vi "mean bulid.vi"(6 "reset data":bool, 8 "mean factor":dbl=-40.0 format="%#_13g", 9 "channel":dbl, 10 "new data":T2, 11 "memory data":T1(array[cluster])) -> (0 "amp cal":cluster{"freqency":dbl[], "Array":dbl[]}, 1 "phase cal":cluster{"freqency":dbl[], "Array":dbl[]}, 3 "memory data":T1(array[cluster]))   [LabVIEW 2021]
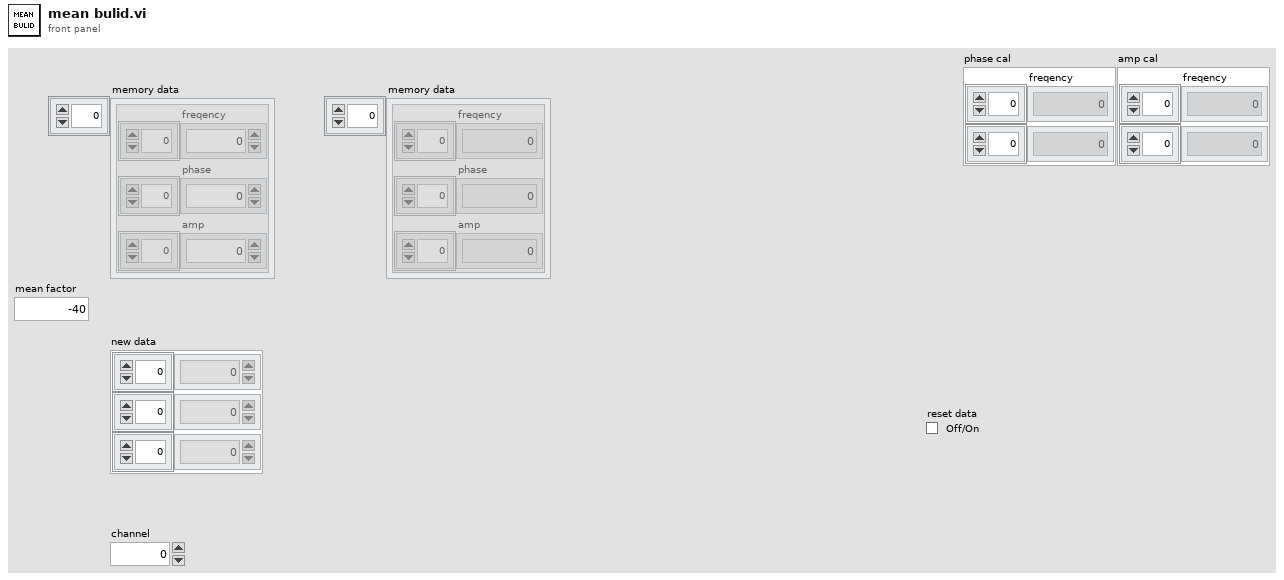
[diagram p1: front panel]
types:
  T1 = cluster{"freqency":dbl[], "phase":dbl[], "amp":dbl[]}[]
  T2 = cluster{"Array":dbl[], "Array":dbl[], "Array":dbl[]}
  T3 = cluster{"freqency":dbl[], "phase":dbl[], "amp":dbl[]}
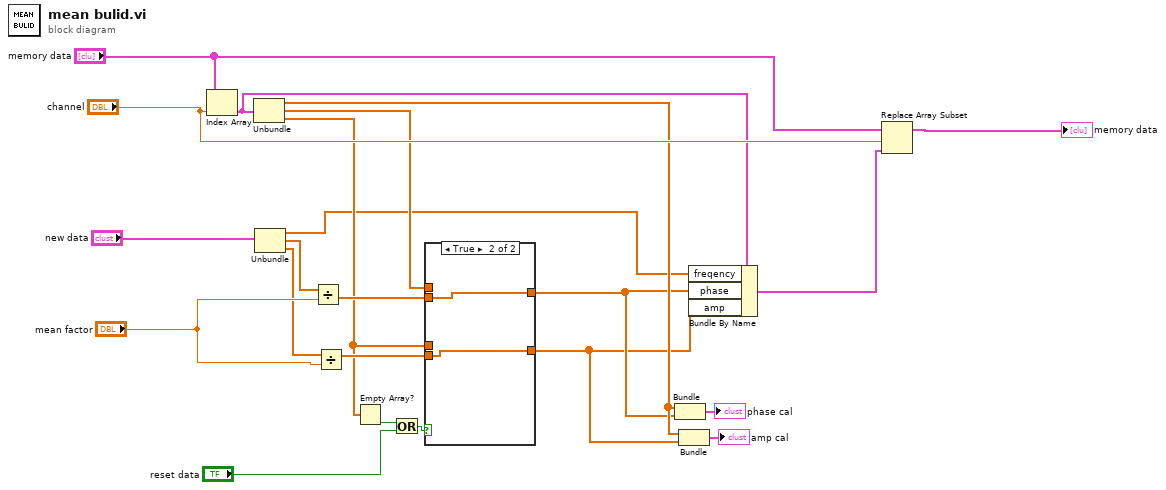
[diagram p0: block diagram]
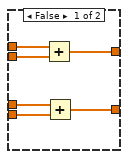
[diagram p2: hidden frame]
diagram:
  n1 = Index Array(array="memory data", index="channel") -> (element=w5:T3)
  n2 = Unbundle(w5) -> ("freqency"=w13:dbl[], "phase"=w18:dbl[], "amp"=w8:dbl[])
  n3 = Unbundle("new data") -> ("Array"=w4:dbl[], "Array"=w20:dbl[], "Array"=w15:dbl[])
  n4 = Divide(x=w20, y="mean factor") -> (x/y=w19:dbl[])
  n5 = Divide(x=w15, y="mean factor") -> (x/y=w17:dbl[])
  n6 = Empty Array?(array=w8) -> (empty?=w3:bool)
  n7 = Or(x=w3, y="reset data") -> (x .or. y?=w1:bool)
  n8 = case shown="True" w1 {
    tunnel: w19 -> [w28 w30]
    tunnel: w18 -> [w27 _]
    tunnel: w17 -> [w26 w29]
    tunnel: [w25 w30] -> w12
    tunnel: [w24 w29] -> w11
    tunnel: w8 -> [w23 _]
    frame False {
      n9 = Add(x=w27, y=w28) -> (x+y=w25:dbl[])
      n10 = Add(x=w23, y=w26) -> (x+y=w24:dbl[])
    }
    frame True {
    }
  }
  n11 = Bundle("freqency"=w13, w12) -> (→"phase cal":cluster{"freqency":dbl[], dbl[]})  [unwired: 1 in]
  n12 = Bundle("freqency"=w13, w11) -> (→"amp cal":cluster{"freqency":dbl[], dbl[]})  [unwired: 1 in]
  n13 = Bundle By Name(cluster=w5, "freqency"=w4, "phase"=w12, "amp"=w11) -> (w7:T3)
  n14 = Replace Array Subset(array="memory data", new element=w7, index="channel") -> (→"memory data":T1)
